vi "closeHDF5.vi"(8 "error in (no error)":errorcluster, 10 "Save Analog Signals":bool=TRUE, 11 "Photodiode in":refnum<class "Photodiode.lvclass">) -> (0 "error out":errorcluster, 3 "Photodiode out":refnum<class "Photodiode.lvclass">)   [LabVIEW 2014, in "Photodiode.lvclass"]
uses:
  Photodiode.lvclass
  Photodiode.lvclass/Photodiode.ctl
  private/HDF5Tools32/LabView/HDF5Tools.lvlib
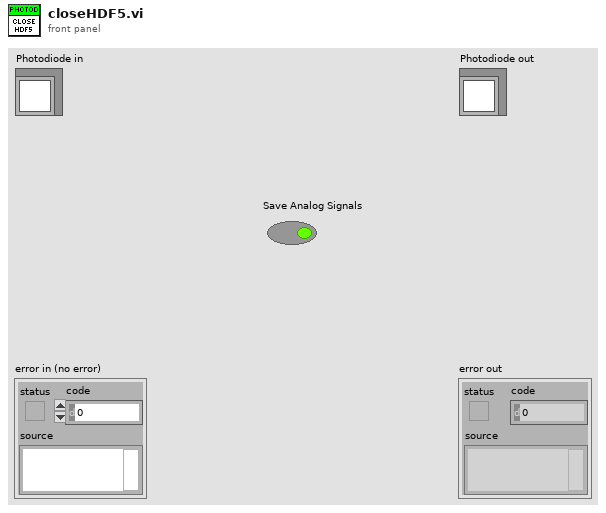
[diagram p1: front panel]
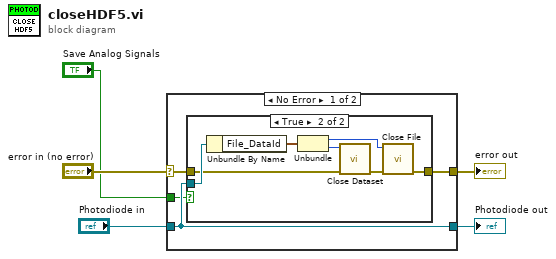
[diagram p0: block diagram]
diagram:
  n1 = case shown="No Error" "error in (no error)" {
    selector: "error in (no error)" -> [w8 w19]
    tunnel: [w7 w19] -> w4
    tunnel: [w9 w18] -> w2
    tunnel: "Photodiode in" -> [w9 w18]
    tunnel: "Save Analog Signals" -> [w6 _]
    frame No Error {
      n2 = case shown="True" w6 {
        tunnel: w9 -> [_ w14]
        tunnel: w8 -> [w10 w12]
        tunnel: [w10 w11] -> w7
        frame False {
        }
        frame True {
          n3 = Unbundle By Name(w14) -> ("File_DataId"=w13:cluster{"file_id":i32, "Dataset id":i32})
          n4 = Unbundle(w13) -> ("file_id"=w15:i32, "Dataset id"=w16:i32)
          n5 = call "Close Dataset.vi"("error in (no error)"=w12, "dataset_id"=w16) -> ("error out"=w17:errorcluster)  [unwired: 9 in]
          n6 = call "Close File.vi"("error in (no error)"=w17, "file_id"=w15) -> ("error out"=w11:errorcluster)  [unwired: 9 in]
        }
      }
    }
    frame Error {
    }
  }
  "error out" <- w4
  "Photodiode out" <- w2
